vi "Interference 1065-366 Textfile.vi"(8 "error in (no error)":errorcluster caption="Fehler (Eingang, kein Fehler)") -> (0 "error out":errorcluster caption="Fehler (Ausgang)", 2 "Tabellen-String":string, 3 "Tabelle für Textdatei":string[](array[string]), 4 "Ergebnis":T1)   [LabVIEW 2020, in "EPA 1065.lvlib" / "HovaCAL Interference verificaton.lvlib"]
uses:
  HovaCAL Interference verificaton.lvlib
  Sprachverwaltung/Sprachverwaltung.lvlib
  Sprachverwaltung/FGV Aktion Tabelle zerlegen.ctl
  Seiten/System Einstellungen V2/Aktioen FGV System Konstanten.ctl
  Seiten/System Einstellungen V2/System Einstellungen V2.lvlib
  Aktion Index uebersetzten.ctl
  Seiten/FT-IR/FGV FT-IR Aktionen.ctl
  Seiten/FT-IR/FT-IR.lvlib
  Aktion FGV Interference.ctl
  Visualisierungs Elemente/String - Ausgabefeld.ctl
  Ergebnis.ctl
panel:
  out "max. Flow Weighted Mean:":T2 caption="%"
  out "Konzentration FlowWeightedMean":sgl=120.0 caption="Concentration:" min=0 format="%#.2f"
  out "Konzentration Komponente":sgl=120.0 caption="Concentration:" min=0
  out "Komponente:":T2 caption="ppm"
  out "[%]":sgl=120.0 caption="Interference:" min=0 format="%#.6g"
  out "Grenze in ppm:":sgl=2.0 min=0 format="%#.6g"
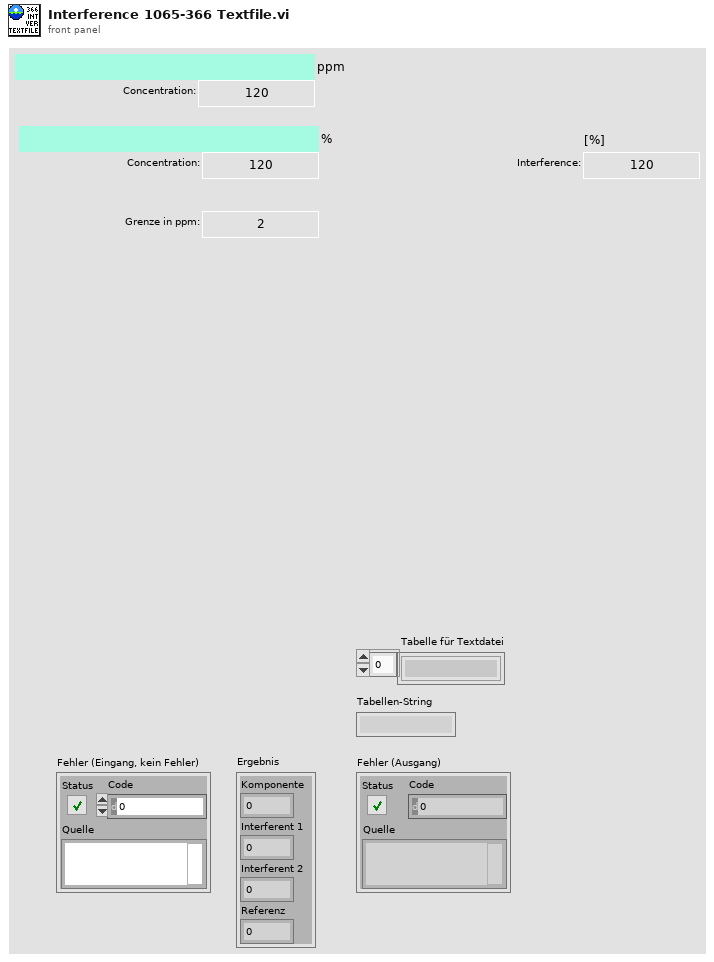
[diagram p1: front panel]
types:
  T1 = typedef "EPA 1065.lvlib/HovaCAL Interference verificaton.lvlib/Ergebnis.ctl" = cluster{"Komponente":sgl, "Interferent 1":sgl, "Interferent 2":sgl, "Referenz":sgl}
  T2 = typedef "String - Ausgabefeld.ctl" = string
  T3 = typedef "System Einstellungen V2.lvlib/Aktioen FGV System Konstanten.ctl" = enum16{"lesen", "laden", "speichern", "Sprache"}
  T4 = typedef "EPA 1065.lvlib/HovaCAL Interference verificaton.lvlib/Aktion Index uebersetzten.ctl" = enum16{"lesen", "schreiben", "auswerten", "Referenzwert", "KompIndex", "RefInterferIndex", "KontrInterfIndex"}
  T5 = typedef "FT-IR.lvlib/FGV FT-IR Aktionen.ctl" = enum16{"lesen", "NOG setzen", "NOS setzen", "Initialisieren", "speichern", "ALLES setzen", "FT-IR Spektrum loggen", "Komm Stoppen", "Spektrum LogKonfig"}
  T6 = typedef "EPA 1065.lvlib/HovaCAL Interference verificaton.lvlib/Aktion FGV Interference.ctl" = enum16{"Lesen", "TestKonfig", "TestSetting", "Einheiten", "Ergebnis", "Laden", "Tabelle", "Speichern", "löschen"}
  T7 = typedef "Sprachverwaltung.lvlib/FGV Aktion Tabelle zerlegen.ctl" = enum16{"laden", "vereinzeln", "speichern"}
  T8 = typedef "EPA 1065.lvlib/HovaCAL Interference verificaton.lvlib/TestSetting.ctl" = cluster{"Bearbeiter:":string, "Pfad:":path, "Textname:":string, "Analysator":T9}
  T9 = typedef "System Einstellungen V2.lvlib/Analysatoren.ctl" = string
  T10 = typedef "EPA 1065.lvlib/HovaCAL Interference verificaton.lvlib/TestKonfig.ctl" = cluster{"TestKonfig H2O":T11, "TestKonfig Interferent":T17}
  T11 = typedef "EPA 1065.lvlib/HovaCAL Interference verificaton.lvlib/TestKonfig H2O.ctl" = cluster{"Modus":T12, "Komponente:":u16, "Eingangs Konzentration:":dbl, "Einheit":T13, "Anzahl Stufen":sgl, "Zeitdauer Stufen":sgl, "Max Fehler":sgl, "zusätzliche Zeitdauer Erster Punkt":sgl, "Punkte umkehren":bool, "Stufen Tabelle":T14, "HovaCAL Flow Input Cluster":T15, "HovaCAL Temperature":T16}
  T12 = typedef "EPA 1065.lvlib/HovaCAL Interference verificaton.lvlib/Modus.ctl" = u16
  T13 = typedef "Linearisierung v2.lvlib/SpanEinstellungen.lvlib/Einheit.ctl" = enum16{"ppm", "%"}
  T14 = typedef "Linearisierung v2.lvlib/Gasteiler.lvlib/Stufen Tabelle.ctl" = string[][]
  T15 = typedef "Linearisierung v2.lvlib/Gasteiler.lvlib/HovaCAL_Interface.lvlib/Controls.lvlib/Flow Einstellung.ctl" = cluster{"HovaCAL Flow Input Cluster":dbl}
  T16 = typedef "Linearisierung v2.lvlib/Gasteiler.lvlib/HovaCAL_Interface.lvlib/Controls.lvlib/Temp Sollwerte Anzeige.ctl" = dbl[]
  T17 = typedef "EPA 1065.lvlib/HovaCAL Interference verificaton.lvlib/TestKonfig Interferents.ctl" = cluster{"MFC1":enum16{"MFC 1"}, "Eingangs Konzentration MFC1":dbl, "Einheit MFC1 Eingang":T13, "Ausgangs Konzentration MFC1":dbl, "Einheit MFC1 Ausgang":T13, "MFC2":T18, "Referenz-Interferent:":u16, "Gasflaschen Nr MFC2":string, "Accuracy MFC2":string, "Eingangs Konzentration MFC2":dbl, "Einheit MFC2 Eingang":T13, "Ausgangs Konzentration MFC2":dbl, "Einheit MFC2 Ausgang":T13, "MFC3":T18, "Kontroll-Interferent:":u16, "Gasflaschen Nr MFC3":string, "Accuracy MFC3":string, "Eingangs Konzentration MFC3":dbl, "Einheit MFC3 Eingang":T13, "Ausgangs Konzentration MFC3":dbl, "Einheit MFC3 Ausgang":T13, "Gasflasche MFC2":T19, "Gasflasche MFC3":T19}
  T18 = typedef "EPA 1065.lvlib/HovaCAL Interference verificaton.lvlib/MFCAuswahl.ctl" = u16
  T19 = typedef "System Einstellungen V2.lvlib/Gasflasche Auswahl.ctl" = u16
  T20 = cluster{"Modell":string, "ProjektNummer":string, "Software Version":string, "Seriennummer":string}
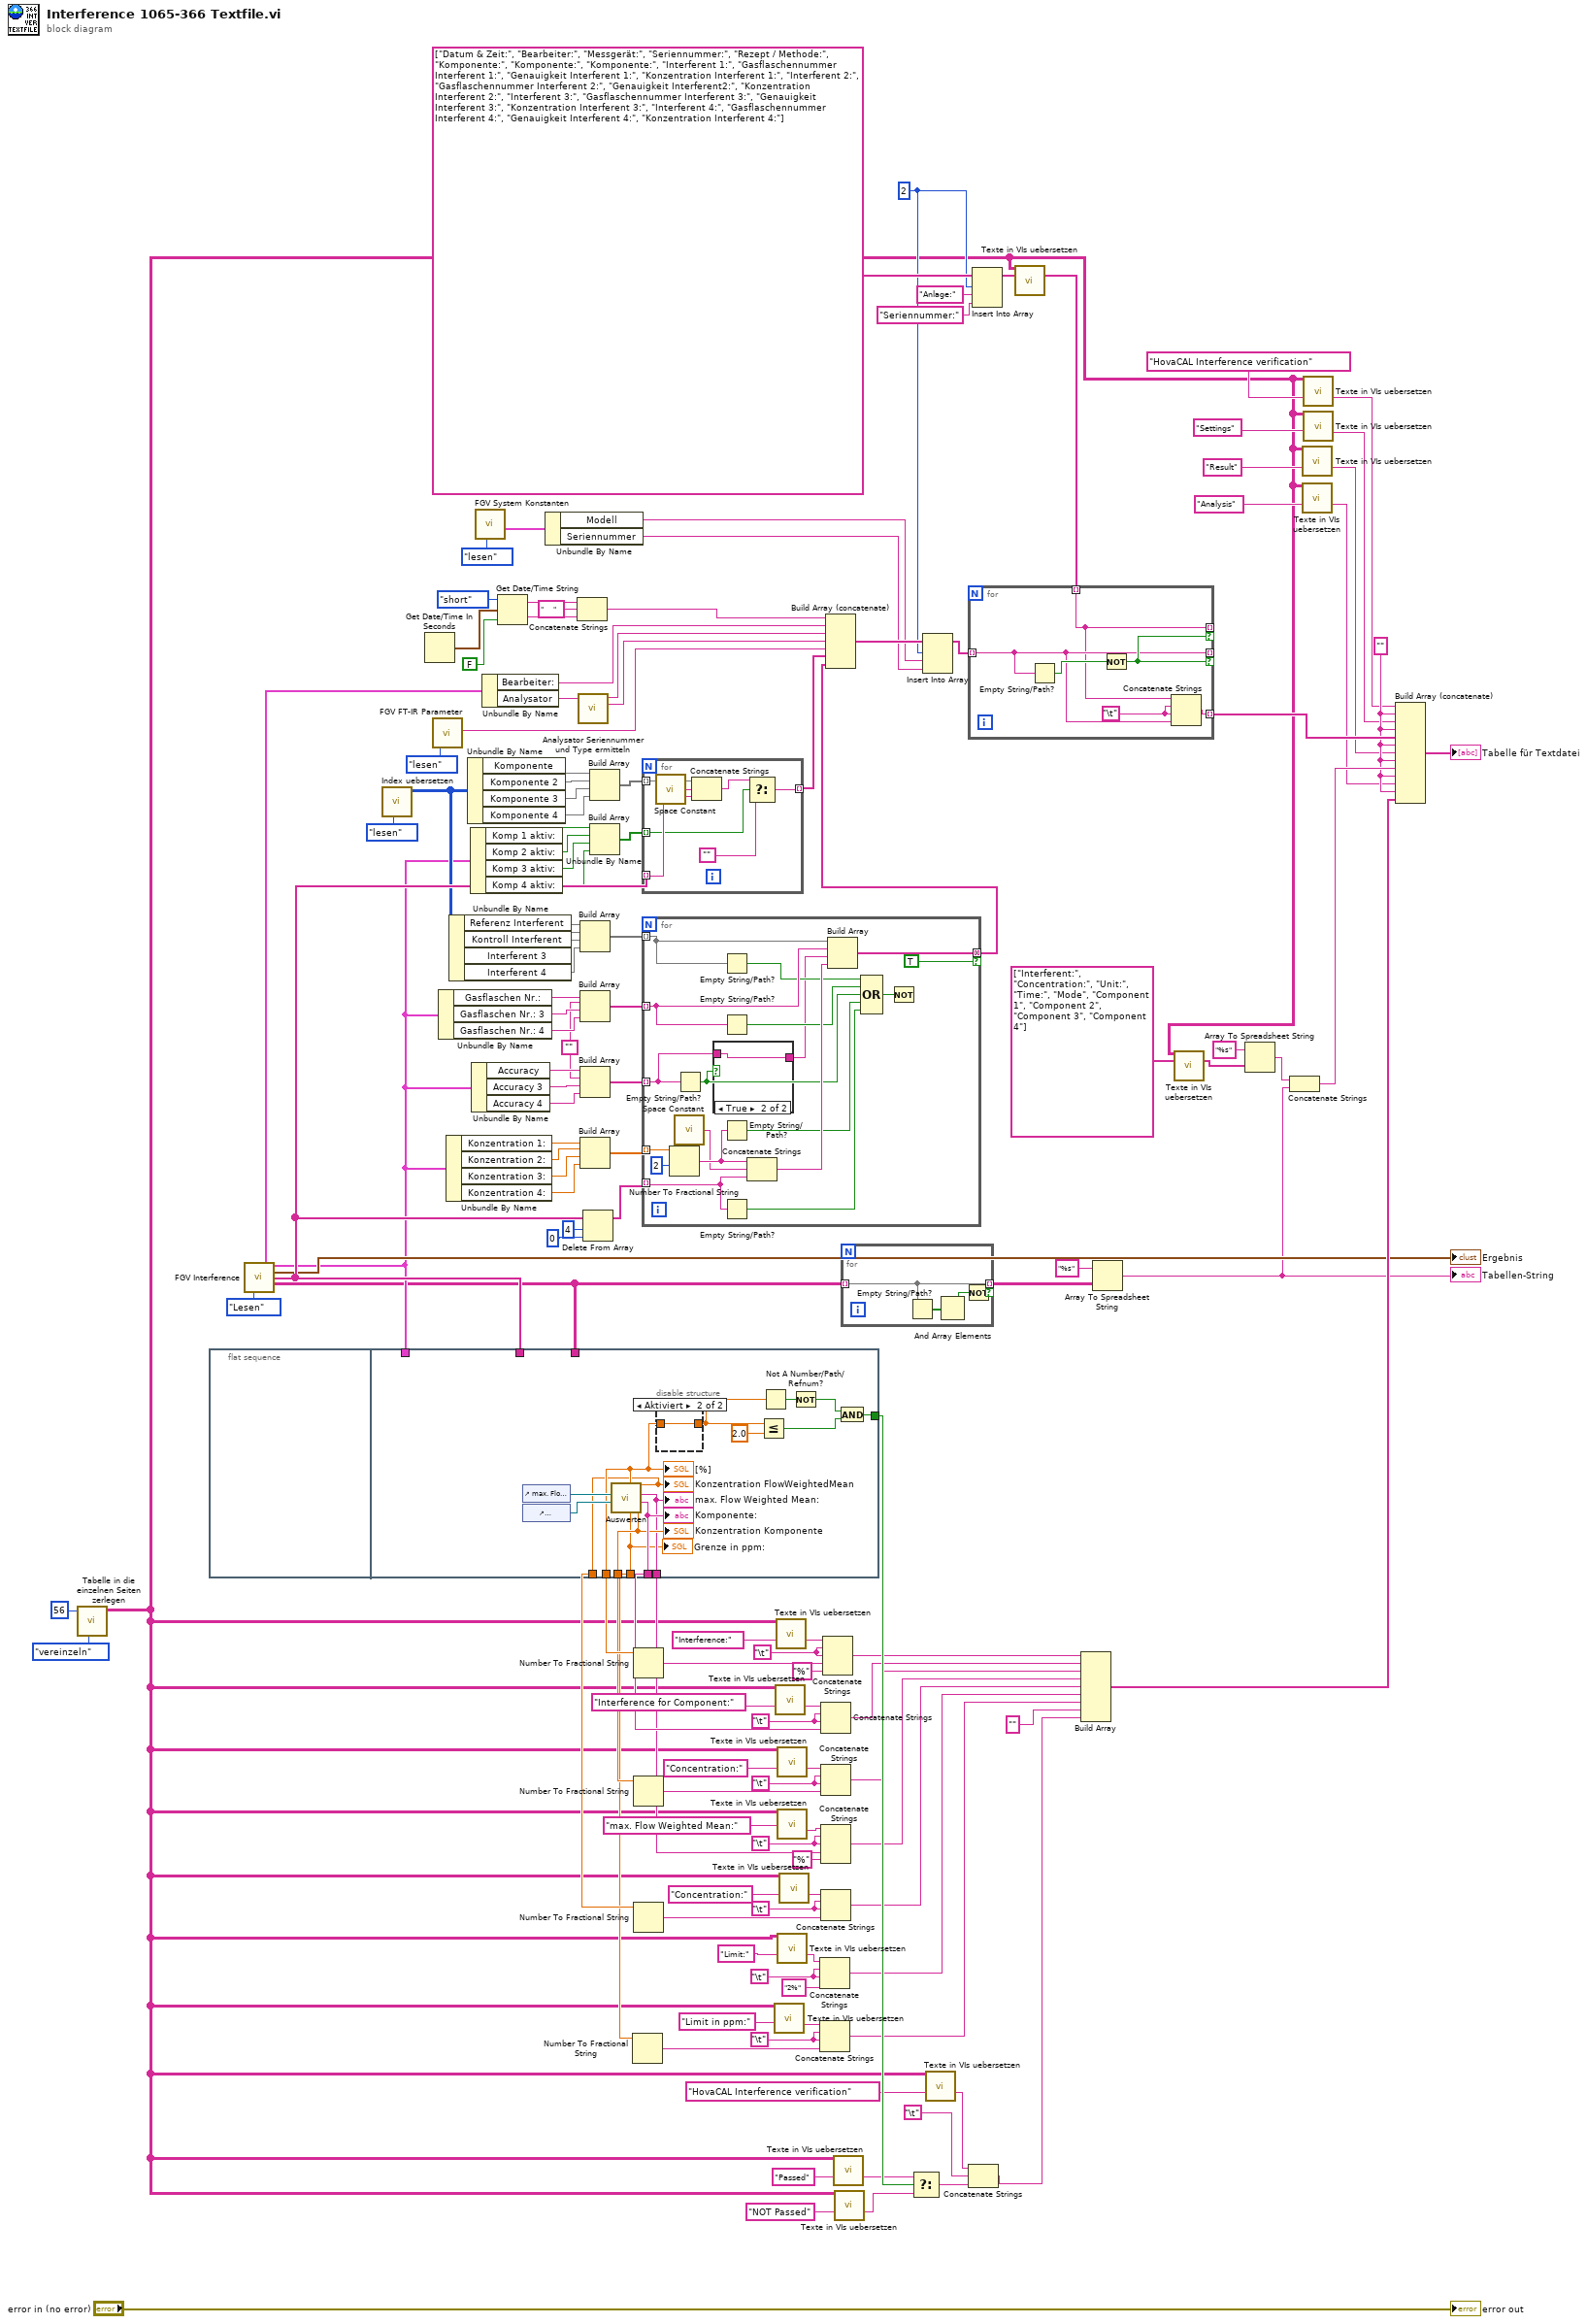
[diagram p0: block diagram]
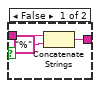
[diagram p2: hidden frame]
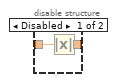
[diagram p3: hidden frame]
diagram:
  w41 = "" ("Element")
  w54 = "\t"
  w55 = "\t"
  w56 = "\t"
  w57 = "\t"
  w58 = "\t"
  w59 = "\t"
  w60 = "\t"
  w82 = ""
  w83 = 2 ("Index")
  n1 = call "Tabelle in die einzelnen Seiten zerlegen.vi"("Aktion"=FGV_Aktion_Tabelle_zerlegen."vereinzeln", "Index (Seite)"=56) -> ("Sprachliste"=w5:string[][])  [unwired: 7 in, 2 out]
  n2 = flat-sequence {
    tunnel: [w150] -> w141
    tunnel: w118 -> [_]
    tunnel: w46 -> [_]
    tunnel: w49 -> [_]
    tunnel: [w149] -> w80
    tunnel: [w148] -> w77
    tunnel: [w147] -> w73
    tunnel: [w146] -> w72
    tunnel: [w145] -> w67
    tunnel: [w144] -> w65
    frame #0 {
    }
    frame #1 {
      n3 = control-ref of="max. Flow Weighted Mean:"() -> (w157:refnum<vi>)
      n4 = control-ref of="Komponente:"() -> (w156:refnum<vi>)
      n5 = call "Auswerten.vi"("Komponente:"=w156, "max. Flow Weighted Mean:"=w157) -> ("Konzentration Komponente"=w147:dbl, "Komponente:"=w148:T2, "max. Flow Weighted Mean:"=w146:T2, "Konzentration FlowWeightedMean"=w145:dbl, "Limit in ppm"=w144:dbl, "[%]"=w149:dbl)  [unwired: 4 in]
      "max. Flow Weighted Mean:" <- w146
      "Konzentration FlowWeightedMean" <- w145
      "Konzentration Komponente" <- w147
      "Komponente:" <- w148
      "[%]" <- w149
      "Grenze in ppm:" <- w144
      n6 = disable-structure shown="Aktiviert" {
        disable-tunnel: [w159 w160] -> w154
        disable-tunnel: w149 -> [w158 w160]
        frame Disabled {
          n7 = Absolute Value(x=w158) -> (abs(x)=w159:dbl)
        }
        frame Enabled {
        }
      }
      n8 = Less Or Equal?(x=w154, y=2.0) -> (x <= y?=w152:bool)
      n9 = Not A Number/Path/Refnum?(number/path/refnum=w154) -> (NaN/Path/Refnum?=w153:bool)
      n10 = Not(x=w153) -> (.not. x?=w151:bool)
      n11 = And(x=w151, y=w152) -> (x .and. y?=w150:bool)
    }
  }
  n12 = call "FGV Interference.vi"("Aktion FGV Interference"=Aktion_FGV_Interference."Lesen") -> ("TestSetting"=w139:T8, "TestKonfig"=w49:T10, "Ergebnis"=→"Ergebnis":T1, "Einheiten"=w118:string[], "Tabelle"=w46:T2[][])  [unwired: 9 in, 1 out]
  n13 = call "Index uebersetzen.vi"("Aktion"=Aktion_Index_uebersetzten."lesen") -> ("Index Array out"=w112:i32[][])  [unwired: 5 in, 5 out]
  n14 = Get Date/Time In Seconds() -> (seconds since 1Jan1904=w138:timestamp)
  n15 = call "FGV FT-IR Parameter.vi"("Aktion"=FGV_FT-IR_Aktionen."lesen") -> ("Current Recipe"=w119:string)  [unwired: 11 in, 7 out]
  n16 = Unbundle By Name(w49) -> ("Gasflaschen Nr.:"=w111:string, "Gasflaschen Nr.: 3"=w110:string, "Gasflaschen Nr.: 4"=w109:string)
  n17 = Unbundle By Name(w49) -> ("Konzentration 1:"=w108:dbl, "Konzentration 2:"=w107:dbl, "Konzentration 3:"=w106:dbl, "Konzentration 4:"=w105:dbl)
  n18 = Unbundle By Name(w112) -> ("Referenz Interferent"=w116, "Kontroll Interferent"=w115, "Interferent 3"=w114, "Interferent 4"=w113)
  n19 = Unbundle By Name(w112) -> ("Komponente"=w130, "Komponente 2"=w129, "Komponente 3"=w128, "Komponente 4"=w39)
  n20 = Unbundle By Name(w49) -> ("Komp 1 aktiv:"=w127:bool, "Komp 2 aktiv:"=w126:bool, "Komp 3 aktiv:"=w125:bool, "Komp 4 aktiv:"=w38:bool)
  n21 = Unbundle By Name(w49) -> ("Accuracy"=w98:string, "Accuracy 3"=w97:string, "Accuracy 4"=w96:string)
  n22 = call "FGV System Konstanten.vi"("Aktionen"=Aktioen_FGV_System_Konstanten."lesen") -> ("Cluster out"=w91:T20)  [unwired: 6 in, 4 out]
  n23 = Unbundle By Name(w139) -> ("Bearbeiter:"=w121:string, "Analysator"=w4:T9)
  n24 = Get Date/Time String(date format (0)=enum16{"short", "long", "abbreviated"}."short" ("Datumsformat (0)"), seconds (now)=w138, want seconds? (F)=FALSE ("Angabe von Sekunden? (F)")) -> (date string=w137:string, time string=w136:string)
  n25 = Unbundle By Name(w91) -> ("Modell"=w87:string, "Seriennummer"=w86:string)
  n26 = Concatenate Strings(w137, "     " ("String"), w136) -> (w122:string)
  n27 = call "Analysator Seriennummer und Type ermitteln.vi"("Analysator"=w4) -> ("Type"=w3:string, "Name für Protokoll"=w2:string)  [unwired: 8 in, 1 out]
  n28 = Build Array(w116, w115, w114, w113) -> (w104:void[])
  n29 = Build Array(w111, w82, w110, w109) -> (w103:string[])
  n30 = Build Array(w98, w82, w97, w96) -> (w95:string[])
  n31 = Build Array(w108, w107, w106, w105) -> (w102:dbl[])
  n32 = Delete From Array(array=w118, length=4 ("Länge"), index=0 ("Index")) -> (array with subset deleted=w100:string[])  [unwired: 1 out]
  n33 = Build Array(w130, w129, w128, w39) -> (w124:void[])
  n34 = Build Array(w127, w126, w125, w38) -> (w123:bool[])
  n35 = Number To Fractional String(number=w65) -> (F-format string=w66:string)  [unwired: 3 in]
  n36 = Number To Fractional String(number=w80) -> (F-format string=w81:string)  [unwired: 3 in]
  n37 = Number To Fractional String(number=w73) -> (F-format string=w74:string)  [unwired: 3 in]
  n38 = Number To Fractional String(number=w67) -> (F-format string=w68:string)  [unwired: 3 in]
  n39 = for {
    tunnel: [w164] -> w120 mode=indexing
    tunnel: w124 -> [w167] mode=indexing
    tunnel: w123 -> [w163] mode=indexing
    tunnel: w118 -> [w166] mode=indexing
    n40 = call <vilib>:"Space Constant.vi"() -> ("String"=w165:string)
    n41 = Concatenate Strings(w167, w165, w166) -> (w162:string)
    n42 = Select(t=w162, s=w163, f="") -> (s? t:f=w164:string)
  }
  n43 = for {
    tunnel: w104 -> [w182] mode=indexing
    tunnel: w103 -> [w181] mode=indexing
    tunnel: w102 -> [w185] mode=indexing
    tunnel: w100 -> [w184] mode=indexing
    tunnel: [w179] -> w99 mode=concatenating if=TRUE
    tunnel: w95 -> [w169] mode=indexing
    n44 = Number To Fractional String(number=w185, precision (6)=i16 2 ("Genauigkeit (6)")) -> (F-format string=w183:string)  [unwired: 2 in]
    n45 = call <vilib>:"Space Constant.vi"() -> ("String"=w173:string)
    n46 = Empty String/Path?(string/path=w169) -> (empty?=w168:bool)
    n47 = case shown="True" w168 {
      tunnel: [w187 w189] -> w172
      tunnel: w169 -> [w186 w189]
      frame False {
        n48 = Concatenate Strings(w186, "%" ("String")) -> (w187:string)
      }
      frame True {
      }
    }
    n49 = Empty String/Path?(string/path=w182) -> (empty?=w178:bool)
    n50 = Empty String/Path?(string/path=w181) -> (empty?=w177:bool)
    n51 = Empty String/Path?(string/path=w183) -> (empty?=w174:bool)
    n52 = Empty String/Path?(string/path=w184) -> (empty?=w176:bool)
    n53 = Concatenate Strings(w183, w173, w184) -> (w180:string)
    n54 = Build Array(w182, w181, w172, w180) -> (w179:string[])
    n55 = Compound Arithmetic op=OR ("Mehrfacharithmetik")(w178, w177, w168, w174, w176) -> (w175:bool)
    n56 = Not(x=w175) -> ()  [unwired: 1 out]
  }
  n57 = call "Texte in VIs uebersetzen.vi"("Sprachliste"=w5, "String zum Übersetzen"="Limit in ppm:" ("String")) -> ("String zum Übersetzen"=w14:string)  [unwired: 9 in, 4 out]
  n58 = call "Texte in VIs uebersetzen.vi"("Sprachliste"=w5, "String zum Übersetzen"="Interference for Component:" ("String")) -> ("String zum Übersetzen"=w24:string)  [unwired: 9 in, 4 out]
  n59 = call "Texte in VIs uebersetzen.vi"("Sprachliste"=w5, "String zum Übersetzen"="Interference:" ("String")) -> ("String zum Übersetzen"=w26:string)  [unwired: 9 in, 4 out]
  n60 = call "Texte in VIs uebersetzen.vi"("Sprachliste"=w5, "String zum Übersetzen"="Concentration:" ("String")) -> ("String zum Übersetzen"=w23:string)  [unwired: 9 in, 4 out]
  n61 = call "Texte in VIs uebersetzen.vi"("Sprachliste"=w5, "String zum Übersetzen"="max. Flow Weighted Mean:" ("String")) -> ("String zum Übersetzen"=w21:string)  [unwired: 9 in, 4 out]
  n62 = call "Texte in VIs uebersetzen.vi"("Sprachliste"=w5, "String zum Übersetzen"="Limit:" ("String")) -> ("String zum Übersetzen"=w17:string)  [unwired: 9 in, 4 out]
  n63 = call "Texte in VIs uebersetzen.vi"("Sprachliste"=w5, "String zum Übersetzen"="Concentration:" ("String")) -> ("String zum Übersetzen"=w19:string)  [unwired: 9 in, 4 out]
  n64 = Concatenate Strings(w17, w54, w54, "2%" ("String")) -> (w52:string)
  n65 = Concatenate Strings(w14, w55, w55, w66) -> (w53:string)
  n66 = Concatenate Strings(w24, w59, w59, w77) -> (w76:string)
  n67 = Concatenate Strings(w23, w58, w58, w74) -> (w75:string)
  n68 = Concatenate Strings(w21, w57, w57, w72, T2 "%" ("String")) -> (w71:string)
  n69 = Concatenate Strings(w19, w56, w56, w68) -> (w69:string)
  n70 = Concatenate Strings(w26, w60, w60, w81, "%" ("String")) -> (w78:string)
  n71 = Build Array (concatenate)(w122, w121, w2, w3, w119, w120, w99) -> (w89:string[])
  n72 = call "Texte in VIs uebersetzen.vi"("Sprachliste"=w5, "String zum Übersetzen"=T2 "Passed" ("String")) -> ("String zum Übersetzen"=w10:string)  [unwired: 9 in, 4 out]
  n73 = call "Texte in VIs uebersetzen.vi"("Sprachliste"=w5, "String zum Übersetzen"=T2 "NOT Passed" ("String")) -> ("String zum Übersetzen"=w8:string)  [unwired: 9 in, 4 out]
  n74 = for {
    tunnel: w46 -> [w193] mode=indexing
    tunnel: [w193] -> w45 mode=indexing if=w190
    n75 = Empty String/Path?(string/path=w193) -> (empty?=w192:bool[])
    n76 = And Array Elements(Boolean array=w192) -> (logical AND=w191:bool)
    n77 = Not(x=w191) -> (.not. x?=w190:bool)
  }
  n78 = Select(t=w10, s=w141, f=w8) -> (s? t:f=w12:string)
  n79 = Insert Into Array(array=w89, index=w83, new element #1=w87, new element #2=w86) -> (w88:string[])
  n80 = call "Texte in VIs uebersetzen.vi"("Sprachliste"=w5, "String zum Übersetzen"="HovaCAL Interference verification") -> ("String zum Übersetzen"=w6:string)  [unwired: 9 in, 4 out]
  n81 = Concatenate Strings(w6, "\t", w12) -> (w13:string)
  n82 = Insert Into Array(array=string[] ["Datum & Zeit:", "Bearbeiter:", "Messgerät:", "Seriennummer:", "Rezept / Methode:", "Komponente:", "Komponente:", "Komponente:", "Interferent 1:", "Gasflaschennummer Interferent 1:", "Genauigkeit Interferent 1:", "Konzentration Interferent 1:", "Interferent 2:", "Gasflaschennummer Interferent 2:", "Genauigkeit Interferent2:", "Konzentration Interferent 2:", "Interferent 3:", "Gasflaschennummer Interferent 3:", "Genauigkeit Interferent 3:", "Konzentration Interferent 3:", "Interferent 4:", "Gasflaschennummer Interferent 4:", "Genauigkeit Interferent 4:", "Konzentration Interferent 4:"], index=w83, new element #1="Anlage:" ("Neues Element/Teil-Array"), new element #2="Seriennummer:" ("Neues Element/Teil-Array")) -> (w90:string[])
  n83 = call "Texte in VIs uebersetzen.vi"("Sprachliste"=w5, "String-Array zum Übersetzen"=w90) -> ("String-Array zum Übersetzen"=w93:string[])  [unwired: 9 in, 4 out]
  n84 = for {
    tunnel: w88 -> [w197] mode=indexing
    tunnel: [w197] -> _ mode=indexing if=w198
    tunnel: [w195] -> _ mode=indexing if=w198
    tunnel: w93 -> [w195] mode=indexing
    tunnel: [w196] -> w63 mode=indexing
    w194 = "\t"
    n85 = Empty String/Path?(string/path=w197) -> (empty?=w199:bool)
    n86 = Not(x=w199) -> (.not. x?=w198:bool)
    n87 = Concatenate Strings(w195, w194, w194, w197) -> (w196:string)
  }
  n88 = Build Array(w78, w76, w75, w71, w69, w52, w53, "" ("Element"), w13) -> (w62:string[])
  n89 = Array To Spreadsheet String(array=w45, 3:"%s" ("Format-String")) -> (spreadsheet string=w43:string)  [unwired: 1 in]
  "Tabellen-String" <- w43
  n90 = call "Texte in VIs uebersetzen.vi"("Sprachliste"=w5, "String-Array zum Übersetzen"=string[] ["Interferent:", "Concentration:", "Unit:", "Time:", "Mode", "Component 1", "Component 2", "Component 3", "Component 4"]) -> ("String-Array zum Übersetzen"=w28:string[])  [unwired: 9 in, 4 out]
  n91 = Array To Spreadsheet String(array=w28, 3:"%s" ("Format-String")) -> (spreadsheet string=w44:string)  [unwired: 1 in]
  n92 = Concatenate Strings(w44, w43) -> (w42:string)
  n93 = call "Texte in VIs uebersetzen.vi"("Sprachliste"=w5, "String zum Übersetzen"="Result" ("Element")) -> ("String zum Übersetzen"=w32:string)  [unwired: 9 in, 4 out]
  n94 = call "Texte in VIs uebersetzen.vi"("Sprachliste"=w5, "String zum Übersetzen"="Analysis" ("Element")) -> ("String zum Übersetzen"=w31:string)  [unwired: 9 in, 4 out]
  n95 = call "Texte in VIs uebersetzen.vi"("Sprachliste"=w5, "String zum Übersetzen"="HovaCAL Interference verification" ("Element")) -> ("String zum Übersetzen"=w36:string)  [unwired: 9 in, 4 out]
  n96 = call "Texte in VIs uebersetzen.vi"("Sprachliste"=w5, "String zum Übersetzen"="Settings" ("Element")) -> ("String zum Übersetzen"=w34:string)  [unwired: 9 in, 4 out]
  n97 = Build Array (concatenate)(w36, w41, w34, w41, w63, w41, w32, w41, w42, w41, w31, w41, w62) -> (→"Tabelle für Textdatei":string[])
  "error out" <- "error in (no error)"
